vi "RobustScaler.vi"(8 "error in (no error)":errorcluster caption="entrée d'erreur (pas d'erreur)", 11 "RobustScaler":T1={"with_centering"=TRUE, "with_scaling"=TRUE, "quantile_range"={"q_min"=25.0, "q_max"=75.0}, "copy"=TRUE}) -> (0 "error out":errorcluster, 3 "RobustScaler.lvclass":refnum<class "RobustScaler.lvclass">)   [LabVIEW 2020]
doc: "Scale features using statistics that are robust to outliers.\n\nThis Scaler removes the median and scales the data according to the quantile range (defaults to IQR: Interquartile Range). The IQR is the range between the 1st quartile (25th quantile) and the 3rd quartile (75th quantile).\n\nCentering and scaling happen independently on each feature by computing the relevant statistics on the samples in the training set. Median and interquartile range are then stored to be used on later data using the transform method.\n\nStandardization of a dataset is a common requirement for many machine learning estimators. Typically this is done by removing the mean and scaling to unit variance. However, outliers can often influence the sample mean / variance in a negative way. In such cases, the median and the interquartile range often give better results.\n\n\nParameters : \n\n- with_centering : boolean, True by default\nIf True, center the data before scaling. This will cause transform to raise an exception when attempted on sparse matrices, because centering them entails building a dense matrix which in common use cases is likely to be too large to fit in memory.\n\n- with_scaling : boolean, True by default\nIf True, scale the data to interquartile range.\n\n- quantile_range : tuple (q_min, q_max), 0.0 < q_min < q_max < 100.0\nDefault: (25.0, 75.0) = (1st quantile, 3rd quantile) = IQR Quantile range used to calculate scale_.\n\n- copy : boolean, optional, default is True\nIf False, try to avoid a copy and do inplace scaling instead. This is not guaranteed to always work inplace; e.g. if the data is not a NumPy array or scipy.sparse CSR matrix, a copy may still be returned.\n\n\nMethods :\n\n- Fit : Compute the median and quantiles to be used for scaling.\n\nParameters : \n\nX : array-like, shape [n_samples, n_features]\nThe data used to compute the median and quantiles used for later scaling along the features axis.\n\n- Fit Transform : Fit to data, then transform it.\n\nFits transformer to X and y with optional parameters fit_params and returns a transformed version of X.\n\nParameters\n\nX : {array-like, sparse matrix, dataframe} of shape (n_samples, n_features)\n\ny : ndarray of shape (n_samples,), default=None\nTarget values.\n\nReturns :\n\nX_new : ndarray array of shape (n_samples, n_features_new)\nTransformed array.\n\n\n- Transform : Center and scale the data.\n\nParameters : \n\nX : {array-like, sparse matrix}\nThe data used to scale along the specified axis."
uses:
  RobustScaler.lvclass
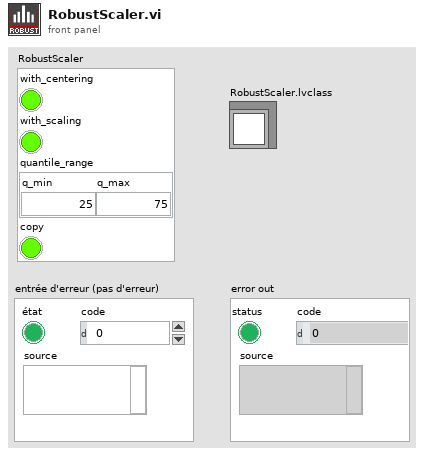
[diagram p1: front panel]
types:
  T1 = cluster{"with_centering":bool, "with_scaling":bool, "quantile_range":cluster{"q_min":dbl, "q_max":dbl}, "copy":bool}
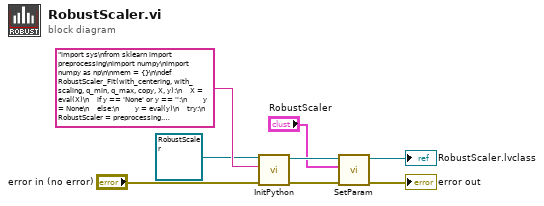
[diagram p0: block diagram]
diagram:
  n1 = call-dynamic "InitPython.vi"("error in (no error)"="error in (no error)", "Python Instruction"="import sys\nfrom sklearn import preprocessing\nimport numpy\nimport numpy as np\n\nmem = {}\n\ndef RobustScaler_Fit(with_centering, with_scaling, q_min, q_max, copy, X, y):\n    X = eval(X)\n    if y == 'None' or y == '':\n        y = None\n    else:\n        y = eval(y)\n    try:\n        RobustScaler = preprocessing.RobustScaler(with_centering, with_scaling, (q_min, q_max), copy).fit(X, y)\n        mem['FitRobustScaler'] = RobustScaler\n        return str('OK')\n    except:\n        erreur = sys.exc_info()\n        typerr = u\"%s\" % (erreur[0])\n        typerr = typerr[typerr.find(\"'\")+1:typerr.rfind(\"'\")]\n        msgerr = u\"%s\" % (erreur[1])\n        message = str('/!\\\\ {0} : {1}'. format(typerr,msgerr))\n        return message \n    \ndef RobustScaler_FitTransform(with_centering, with_scaling, q_min, q_max, copy, X, y):\n    X = eval(X)\n    if y == 'None' or y == '':\n        y = None\n    else:\n        y = eval(y)\n    try:\n        RobustScaler = preprocessing.RobustScaler(with_centering, with_scaling, (q_min, q_max), copy).fit_transform(X, y)\n        dtype = type(RobustScaler)\n        if dtype == numpy.ndarray:\n            RobustScaler = RobustScaler.tolist()\n            return str(RobustScaler) \n        else:\n            Mat = RobustScaler.tocoo()\n            return str(list(zip(Mat.row, Mat.col, Mat.data)))\n    except:\n        erreur = sys.exc_info()\n        typerr = u\"%s\" % (erreur[0])\n        typerr = typerr[typerr.find(\"'\")+1:typerr.rfind(\"'\")]\n        msgerr = u\"%s\" % (erreur[1])\n        message = str('/!\\\\ {0} : {1}'. format(typerr,msgerr))\n        return message \n\ndef RobustScaler_Transform(with_centering, with_scaling, q_min, q_max, copy, X, y):\n    X = eval(X)\n    if y == 'None' or y == '':\n        y = None\n    else:\n        y = eval(y)\n    try:\n        RobustScaler = mem['FitRobustScaler'].transform(X)\n        dtype = type(RobustScaler)\n        if dtype == numpy.ndarray:\n            RobustScaler = RobustScaler.tolist()\n            return str(RobustScaler) \n        else:\n            Mat = RobustScaler.tocoo()\n            return str(list(zip(Mat.row, Mat.col, Mat.data)))\n    except:\n        erreur = sys.exc_info()\n        typerr = u\"%s\" % (erreur[0])\n        typerr = typerr[typerr.find(\"'\")+1:typerr.rfind(\"'\")]\n        msgerr = u\"%s\" % (erreur[1])\n        message = str('/!\\\\ {0} : {1}'. format(typerr,msgerr))\n        return message", "Scikit-learn en entrée"=refnum<class "RobustScaler.lvclass"> refnum ("RobustScaler.lvclass")) -> ("error out"=w3:errorcluster, "Scikit-learn en sortie"=w5:refnum<class "RobustScaler.lvclass">)  [unwired: 7 in]
  n2 = call-dynamic "SetParam.vi"("error in (no error)"=w3, "RobustScaler"="RobustScaler", "RobustScaler.lvclass"=w5) -> ("error out"=→"error out":errorcluster, "RobustScaler.lvclass"=→"RobustScaler.lvclass":refnum<class "RobustScaler.lvclass">)  [unwired: 7 in]
